vi "Get Columns.vi"(8 "error in (no error)":errorcluster, 10 "Table Name":string, 11 "ODBC in":refnum<class "ADODB.lvclass">) -> (0 "error out":errorcluster, 2 "Column Name Array":string[](array[string]), 3 "ODBC out":refnum<class "ADODB.lvclass">)   [LabVIEW 2020, in "ADODB.lvclass"]
uses:
  ADODB.lvclass
  ADODB.lvclass/ADODB.ctl
  <vilib>/addons/database/NI_Database_API.lvlib
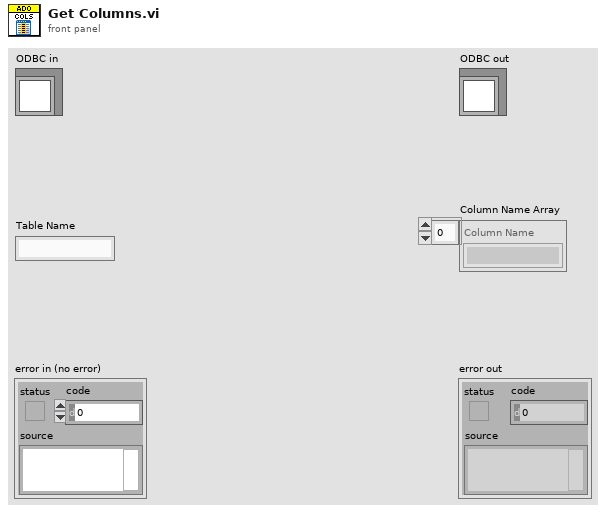
[diagram p1: front panel]
types:
  T1 = typedef "NI_Database_API.lvlib/Conn ObjectReference.ctl" = refnum<k1>
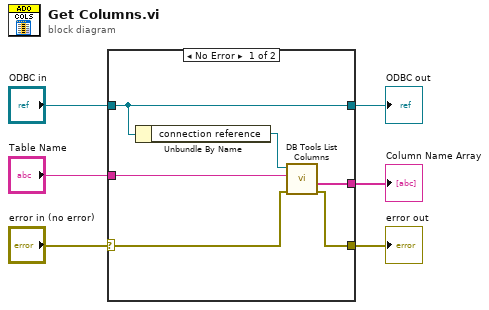
[diagram p0: block diagram]
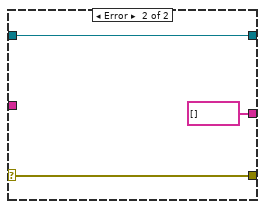
[diagram p2: hidden frame]
diagram:
  n1 = case shown="No Error" "error in (no error)" {
    selector: "error in (no error)" -> [w10 w15]
    tunnel: [w9 w15] -> w5
    tunnel: "ODBC in" -> [w7 w13]
    tunnel: [w7 w13] -> w3
    tunnel: "Table Name" -> [w12 _]
    tunnel: [w11 string[] [] ("columns")] -> w1
    frame No Error {
      n2 = Unbundle By Name(w7) -> ("connection reference"=w8:T1)
      n3 = call <vilib>:"DB Tools List Columns.vi"("error in (no error)"=w10, "table"=w12, "connection reference"=w8) -> ("error out"=w9:errorcluster, "columns"=w11:string[])  [unwired: 1 in, 2 out]
    }
    frame Error {
    }
  }
  "error out" <- w5
  "ODBC out" <- w3
  "Column Name Array" <- w1
